vi "AcquirePlotTime.vi"(10 "重启？":bool) -> (2 "时间":u32)   [LabVIEW 2015, in "Acquisition.lvlib"]
uses:
  Acquisition.lvlib
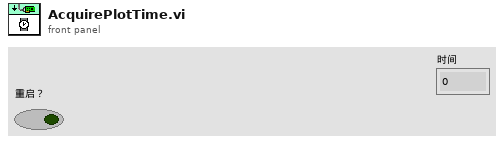
[diagram p1: front panel]
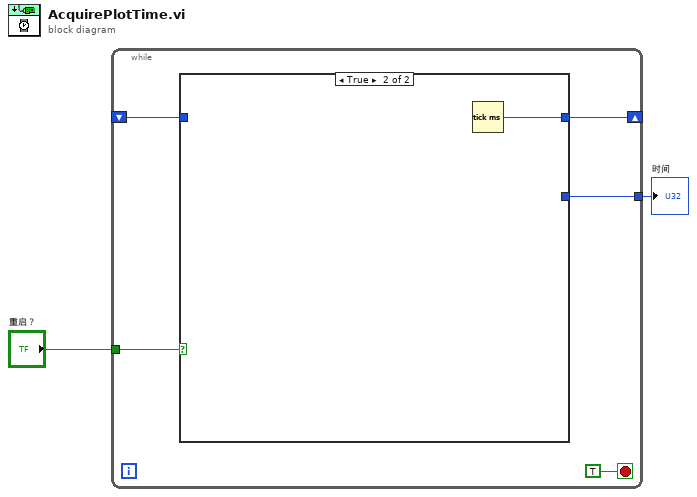
[diagram p0: block diagram]
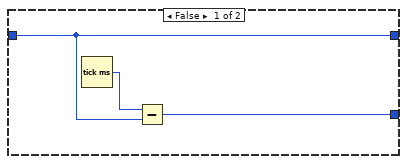
[diagram p2: hidden frame]
diagram:
  n1 = while {
    shift-right: [w6] -> _
    shift-left: _ -> [w5]
    tunnel: "重启？" -> [w7]
    tunnel: [w4] -> w1
    stop <- TRUE stop-if-true
    n2 = case shown="True" w7 {
      tunnel: [w9 w11] -> w6
      tunnel: w5 -> [w9 _]
      tunnel: [w8 _] -> w4
      frame False {
        n3 = Tick Count (ms)() -> (millisecond timer value=w10:u32)
        n4 = Subtract(x=w10, y=w9) -> (x-y=w8:u32)
      }
      frame True {
        n5 = Tick Count (ms)() -> (millisecond timer value=w11:u32)
      }
    }
  }
  "时间" <- w1
